vi "Thermocouple Monitor.vi"() -> ()   [LabVIEW 2013]
uses:
  <vilib>/Utility/file.llb/Write To Spreadsheet File (string).vi
  <vilib>/Utility/file.llb/Write To Spreadsheet File (DBL).vi
panel:
  in  "User":string
  in  "file path (dialog if empty)":path
  in  "DELAY":dbl(knob) scale=0.1..30.0
  in  "stop":bool
  out "Thermocouple Monitor":cluster{dbl[], dbl[]}[](graph)
  out "Temperatures":dbl[](array[numeric])
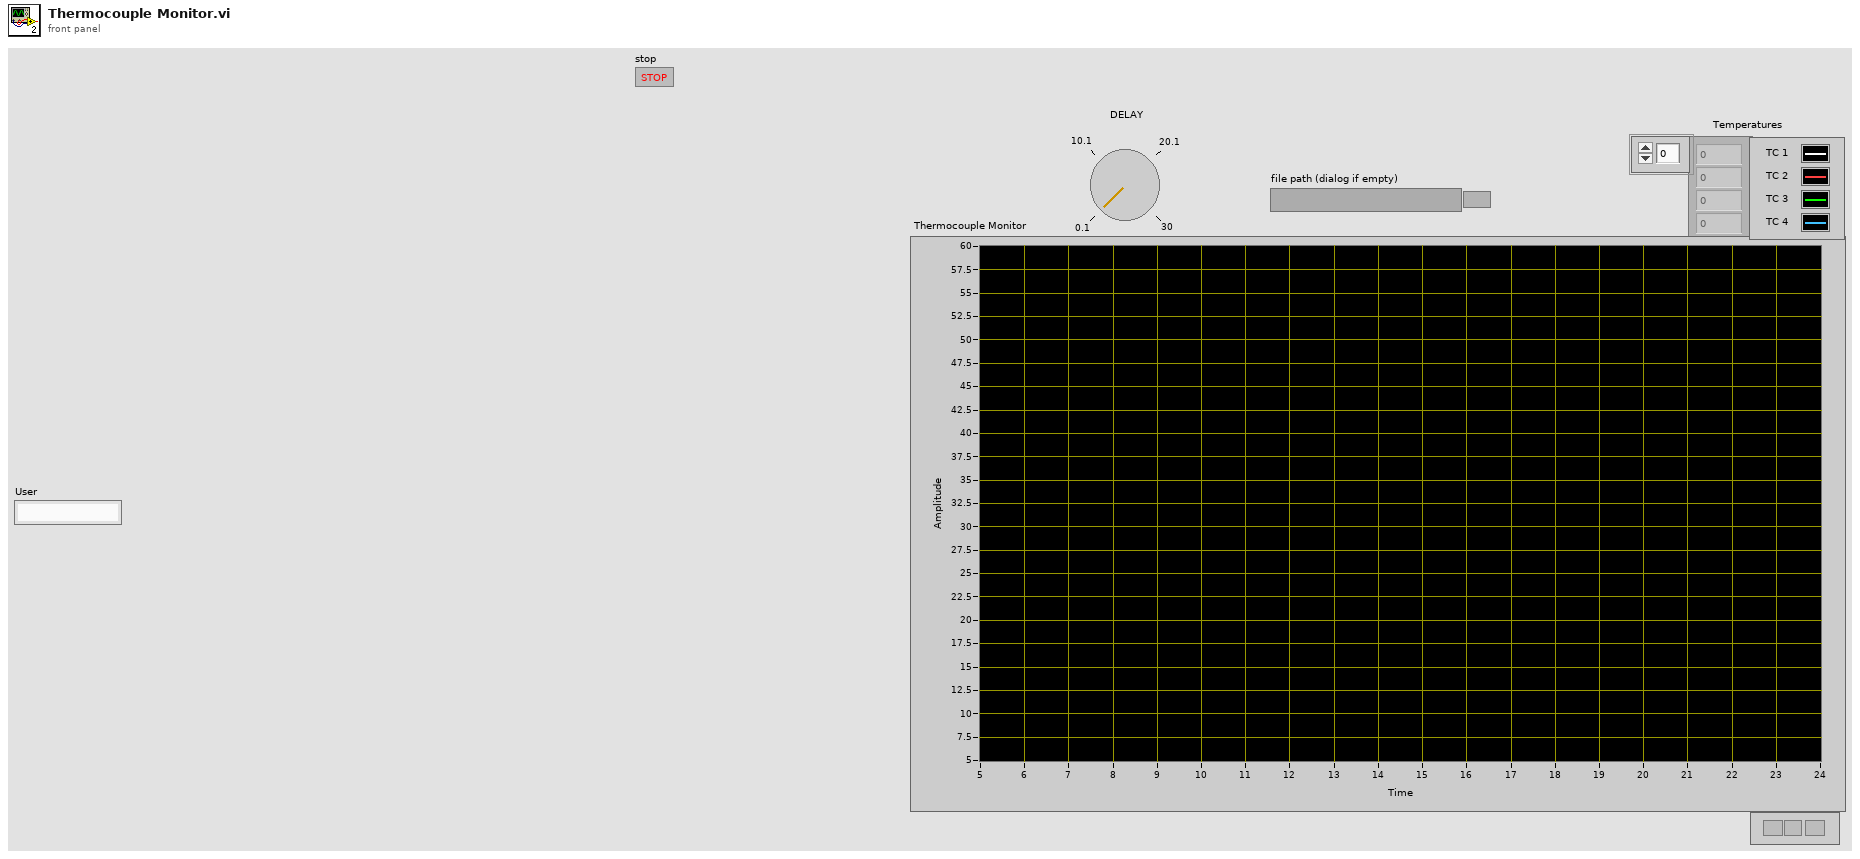
[diagram p1: front panel]
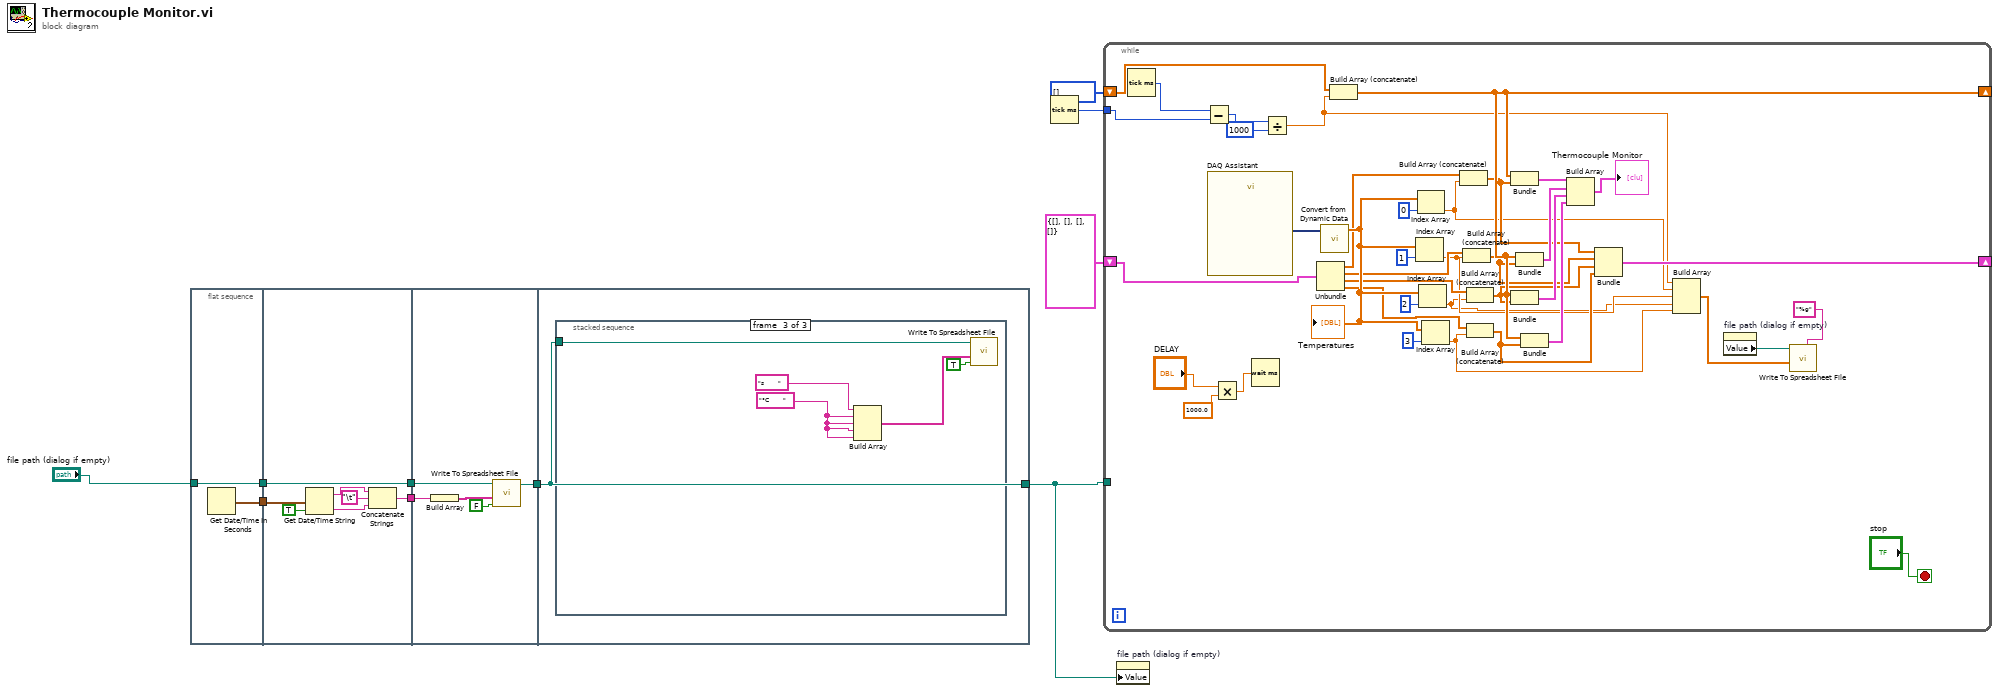
[diagram p0: block diagram]
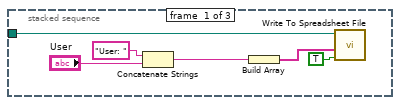
[diagram p2: hidden frame]
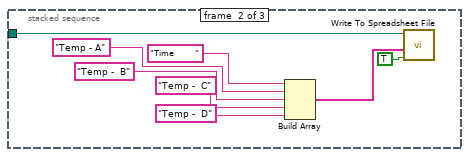
[diagram p3: hidden frame]
diagram:
  n1 = flat-sequence {
    tunnel: [w11] -> w7
    tunnel: [w12] -> w6
    tunnel: "file path (dialog if empty)" -> [w12]
    tunnel: w7 -> [w17]
    tunnel: [w16] -> w5
    tunnel: [w13] -> w4
    tunnel: w6 -> [w13]
    tunnel: w5 -> [w23]
    tunnel: w4 -> [w21]
    tunnel: [w20] -> w3
    tunnel: [w25] -> w1
    tunnel: w3 -> [w25]
    frame #0 {
      n2 = Get Date/Time In Seconds() -> (seconds since 1Jan1904=w11:timestamp)
    }
    frame #1 {
      n3 = Get Date/Time String(seconds (now)=w17, want seconds? (F)=TRUE) -> (date string=w19:string, time string=w15:string)  [unwired: 1 in]
      n4 = Concatenate Strings(w19, "\t", w15) -> (w16:string)
    }
    frame #2 {
      n5 = Build Array(w23) -> (w22:string[])
      n6 = call-poly <vilib>:"Write To Spreadsheet File.vi"("append to file? (new file:F)"=FALSE ("transpose? (no:F)"), "1D data"=w22, "file path (dialog if empty)"=w21) -> ("new file path (Not A Path if cancelled)"=w20:path)  [unwired: 5 in]
    }
    frame #3 {
      n7 = stacked-sequence {
        tunnel: w25 -> [w29 w32 w42]
        frame #0 {
          n8 = Concatenate Strings("User: ", "User") -> (w28:string)
          n9 = Build Array(w28) -> (w30:string[])
          n10 = call-poly <vilib>:"Write To Spreadsheet File.vi"("append to file? (new file:F)"=TRUE ("transpose? (no:F)"), "1D data"=w30, "file path (dialog if empty)"=w29) -> ()  [unwired: 5 in, 1 out]
        }
        frame #1 {
          n11 = Build Array("Time       ", "Temp - A", "Temp -  B" ("element"), "Temp -  C", "Temp -  D") -> (w36:string[])
          n12 = call-poly <vilib>:"Write To Spreadsheet File.vi"("append to file? (new file:F)"=TRUE ("transpose? (no:F)"), "1D data"=w36, "file path (dialog if empty)"=w32) -> ()  [unwired: 5 in, 1 out]
        }
        frame #2 {
          w40 = "°C       "
          n13 = Build Array("s       ", w40, w40, w40, w40) -> (w43:string[])
          n14 = call-poly <vilib>:"Write To Spreadsheet File.vi"("append to file? (new file:F)"=TRUE ("transpose? (no:F)"), "1D data"=w43, "file path (dialog if empty)"=w42) -> ()  [unwired: 5 in, 1 out]
        }
      }
    }
  }
  n15 = Tick Count (ms)() -> (millisecond timer value=w10:u32)
  n16 = while {
    tunnel: w10 -> [w59]
    shift-right: [w77] -> _
    shift-left: u32[] [] -> [w78]
    shift-right: [w66] -> _
    shift-left: cluster{dbl[], dbl[], dbl[], dbl[]} {[], [], [], []} -> [w65]
    tunnel: w1 -> [_]
    stop <- "stop" stop-if-true
    n17 = Tick Count (ms)() -> (millisecond timer value=w60:u32)
    n18 = Subtract(x=w60, y=w59) -> (x-y=w58:u32)
    n19 = call "DAQ Assistant"() -> ("data"=w53:dynamicdata)  [unwired: 17 in, 2 out]
    n20 = Multiply(x="DELAY", y=1000.0) -> (x*y=w56:dbl)
    n21 = Wait (ms)(milliseconds to wait=w56) -> ()  [unwired: 1 out]
    n22 = Divide(x=w58, y=u32 1000) -> (x/y=w52:dbl)
    n23 = Unbundle(w65) -> (w64:dbl[], w63:dbl[], w62:dbl[], w61:dbl[])
    n24 = call "Convert from Dynamic Data"("Dynamic Data Type"=w53) -> ("Array"=w83:dbl[])  [unwired: 3 in]
    "Temperatures" <- w83
    n25 = Build Array (concatenate)(w78, w52) -> (w77:dbl[])
    n26 = Index Array(array=w83, index=1) -> (element=w50:dbl)
    n27 = Index Array(array=w83, index=0) -> (element=w51:dbl)
    n28 = Index Array(array=w83, index=2) -> (element=w49:dbl)
    n29 = Index Array(array=w83, index=3) -> (element=w48:dbl)
    n30 = Build Array (concatenate)(w64, w51) -> (w70:dbl[])
    n31 = Build Array (concatenate)(w63, w50) -> (w69:dbl[])
    n32 = Build Array (concatenate)(w62, w49) -> (w68:dbl[])
    n33 = Build Array (concatenate)(w61, w48) -> (w67:dbl[])
    n34 = Bundle(w77, w70) -> (w76:cluster{dbl[], dbl[]})  [unwired: 1 in]
    n35 = Bundle(w77, w68) -> (w74:cluster{dbl[], dbl[]})  [unwired: 1 in]
    n36 = Bundle(w77, w69) -> (w75:cluster{dbl[], dbl[]})  [unwired: 1 in]
    n37 = Bundle(w77, w67) -> (w73:cluster{dbl[], dbl[]})  [unwired: 1 in]
    n38 = Build Array(w76, w75, w74, w73) -> (→"Thermocouple Monitor":cluster{dbl[], dbl[]}[])
    n39 = Bundle(w70, w69, w68, w67) -> (w66:cluster{dbl[], dbl[], dbl[], dbl[]})  [unwired: 1 in]
    n40 = Build Array(w52, w51, w50, w49, w48) -> (w47:dbl[])
    n41 = property on="file path (dialog if empty)" class="Path"() -> ("Value"=w45:path)  [unwired: 2 in, 2 out]
    n42 = call-poly <vilib>:"Write To Spreadsheet File.vi"("format (%.3f)"="%g", "1D data"=w47, "file path (dialog if empty)"=w45) -> ()  [unwired: 5 in, 1 out]
  }
  n43 = property on="file path (dialog if empty)" class="Path"("Value"=w1) -> ()  [unwired: 2 in, 2 out]
